vi "Main.vi"(7 "mode":T1) -> ()   [LabVIEW 2020, in "InstrumentStudioPlugin.lvlib"]
doc: "This template is for the Queued Message Handler design pattern.\n\nThe Event Handling Loop generates messages based on user interface actions.\n\nThe Message Handling Loop processes messages generated by the Event Handling Loop, or by other messages. The messages are string values, so new messages can be added easily to the Message Cases case structure in the Message Handling Loop. Each message cluster can also provide an optional value for Message Data, which is a variant that can be converted to whatever message-specific data is required."
uses:
  InstrumentStudioPlugin.lvlib
  controls/Plugin Mode.ctl
  InstrumentStudioPluginSDK.lvlibp/Plugin Events Enum.ctl
  controls/Configuration.ctl
  controls/Data.ctl
  Measurement Client Wrapper/Measurement Client Wrapper.lvclass
  controls/UI References.ctl
  Measurement Client Wrapper/Measurement Client Wrapper.lvclass/Measurement Client Wrapper.ctl
  Measurement Client Wrapper/Property/Read Display Name.vi
  Measurement Client Wrapper/Property/Read Version.vi
  subVIs/Message Queue/Enqueue Message (Single).vi
  subVIs/Message Queue/Enqueue Message (Array).vi
  <vilib>/Utility/error.llb/Error Cluster From Error Code.vi
  InstrumentStudioPluginSDK.lvlibp/Read Run Time Configuration.vi
  InstrumentStudioPluginSDK.lvlibp/Read Edit Time Configuration.vi
  InstrumentStudioPluginSDK.lvlibp/Write Run Time Configuration.vi
  InstrumentStudioPluginSDK.lvlibp/Write Edit Time Configuration.vi
  <vilib>/ErrorRing/Error Ring.xnode
  subVIs/Message Queue/Message Queue.lvlib
  subVIs/User Event - Stop/User Event - Stop.lvlib
  InstrumentStudioPluginSDK.lvlibp/Plugin Session.lvclass
  InstrumentStudioPluginSDK.lvlibp
panel:
  in  "Run Measurement":bool
  out "Version":string
  out "Measurement Name":string
  out "Status":string
  in  "Read Run Time Config":bool
  in  "Read Edit Time Config":bool
  in  "Session Id":u64
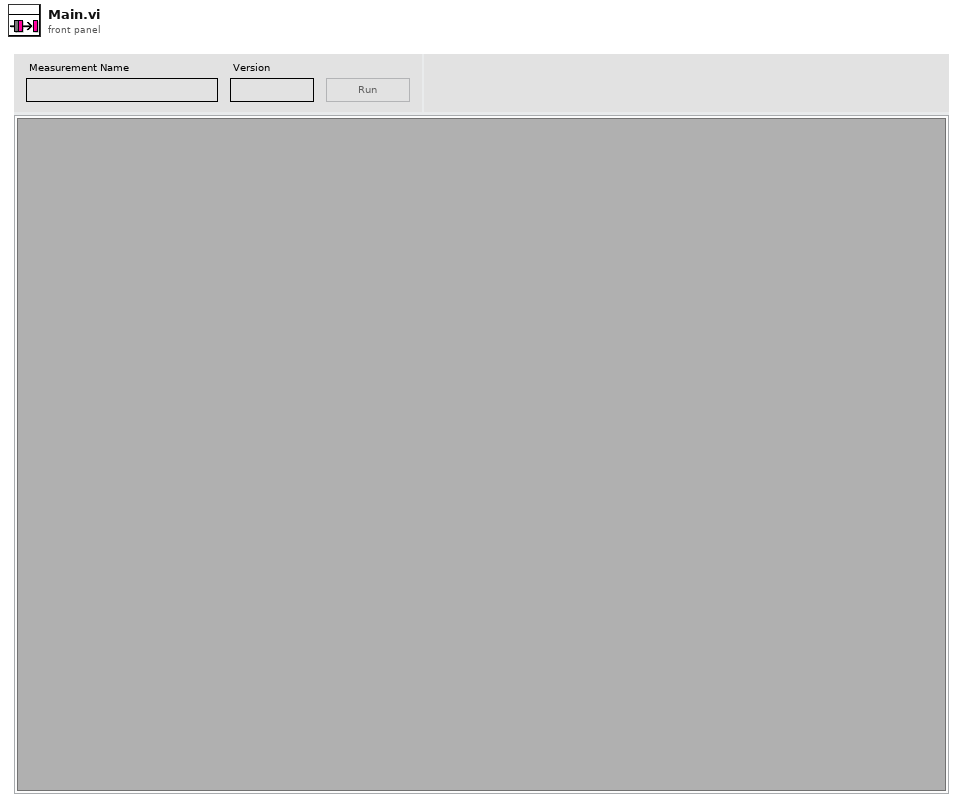
[diagram p1: front panel]
types:
  T1 = typedef "InstrumentStudioPlugin.lvlib/Plugin Mode.ctl" = enum16{"Interactive", "Automated"}
  T2 = typedef "InstrumentStudioPlugin.lvlib/UI References.ctl" = cluster{"UI Subpanel":refnum<vi>, "Status Message":string, "Matching UI & Meas Parameters?":bool}
  T3 = typedef "InstrumentStudioPlugin.lvlib/Data.ctl" = cluster{"Measurement Address":string, "Measurement Port":string, "Measurement Name":string, "Measurement Service":string, "Discovery Service address":string, "Measurement Service [obj]":refnum<class "Measurement Client Wrapper.lvclass">}
  T4 = typedef "InstrumentStudioPlugin.lvlib/Configuration.ctl" = cluster{"sample string":string}
  T5 = typedef "InstrumentStudioPluginSDK.lvlibp/Plugin Events Enum.ctl" = enum16{"Shutdown", "Project Saved", "Stop All Outputs"}
  T6 = typedef "InstrumentStudioPluginSDK.lvlibp/Event Registration Refnum.ctl" = refnum<event-registration>
  T7 = typedef "Message Queue.lvlib/All Message Queues.ctl" = cluster{"UI":refnum<queue>}
  T8 = cluster{"Event Refnum":T6, "Event Registration Refnum":refnum<event-registration>}
  T9 = enum8{"Enabled", "Disabled", "Disabled and Grayed Out"}
  T10 = cluster{"Measurement Name":string, "Measurement Service":string}
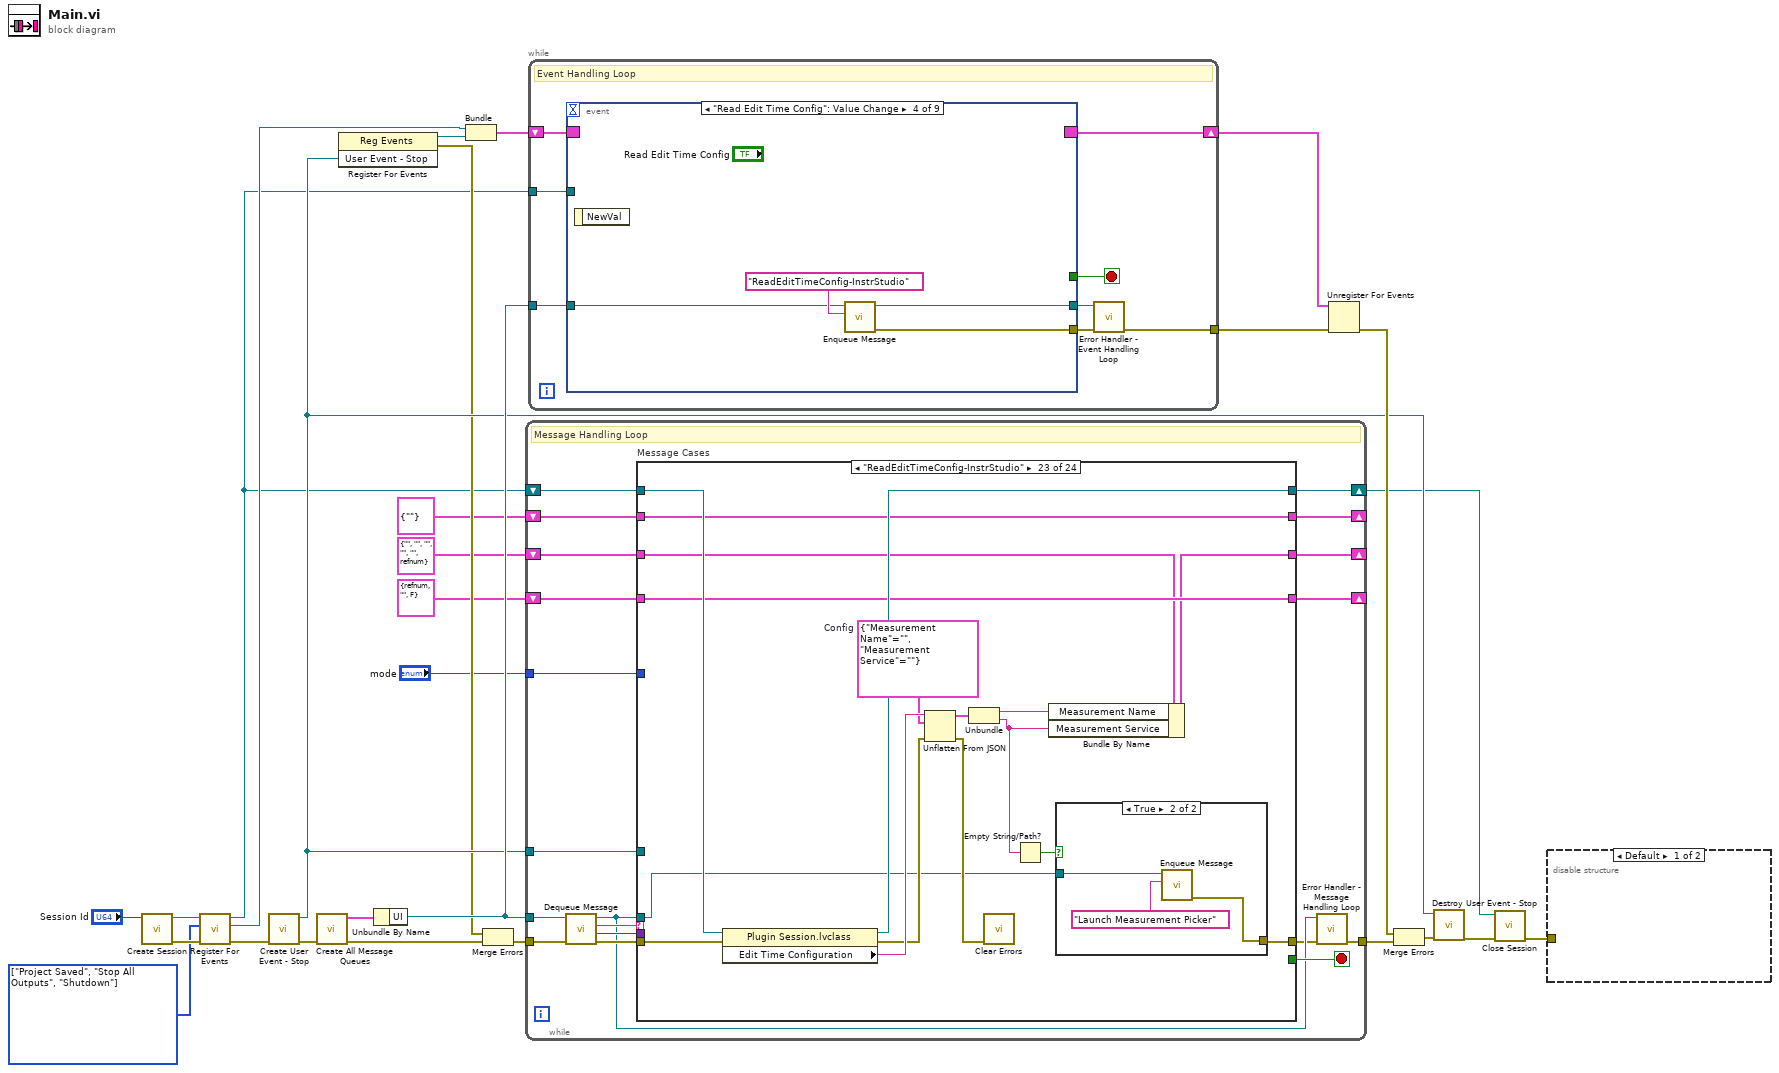
[diagram p0: block diagram]
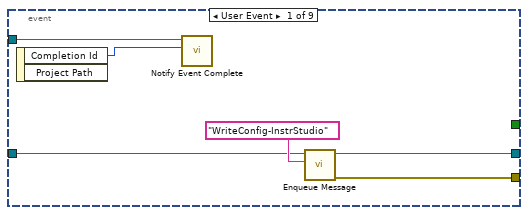
[diagram p3: hidden frame]
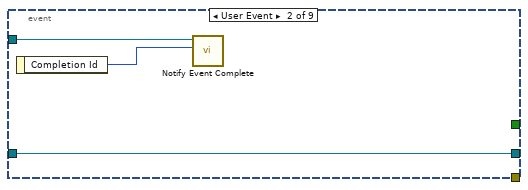
[diagram p4: hidden frame]
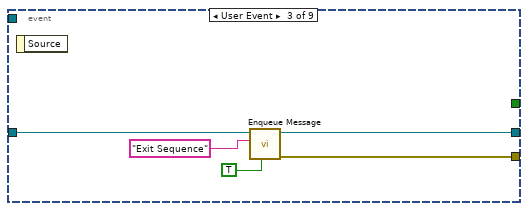
[diagram p5: hidden frame]
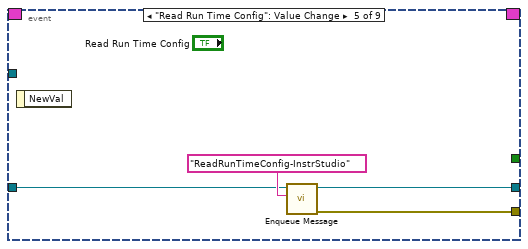
[diagram p6: hidden frame]
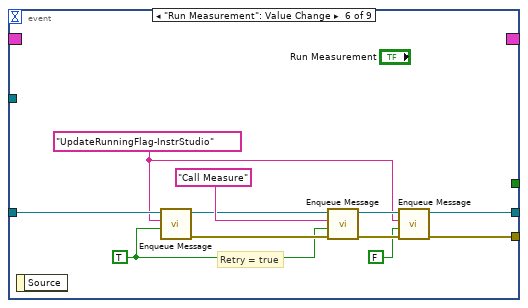
[diagram p7: hidden frame]
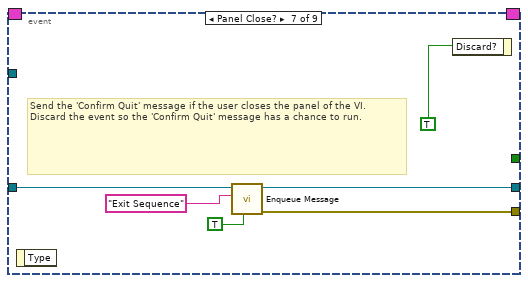
[diagram p8: hidden frame]
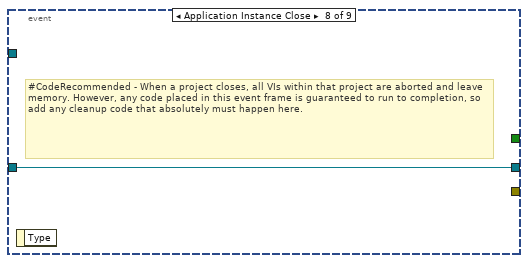
[diagram p9: hidden frame]
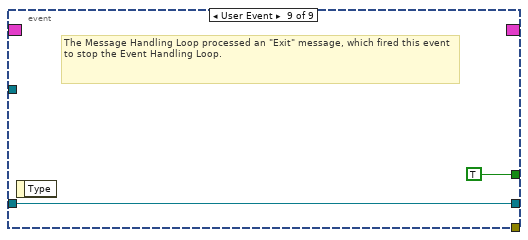
[diagram p10: hidden frame]
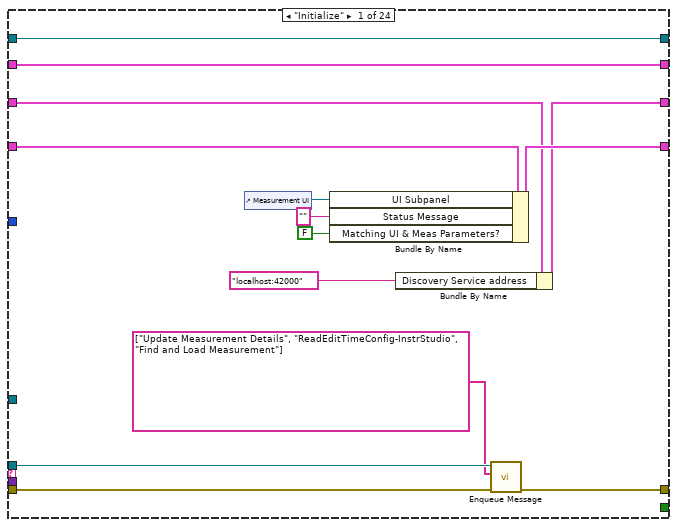
[diagram p11: hidden frame]
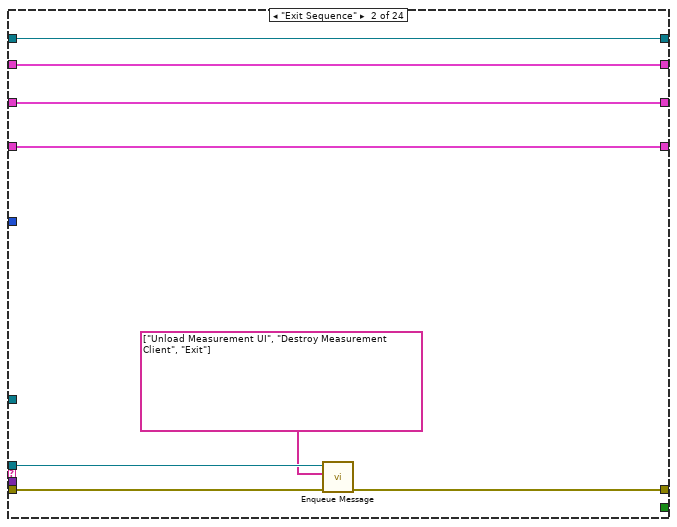
[diagram p12: hidden frame]
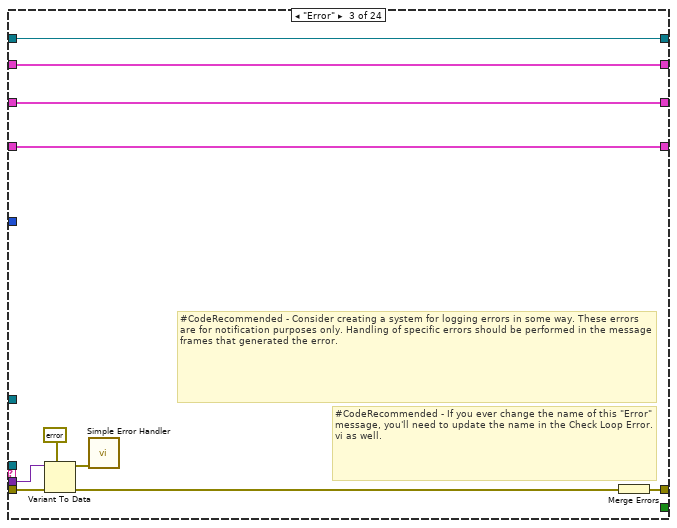
[diagram p13: hidden frame]
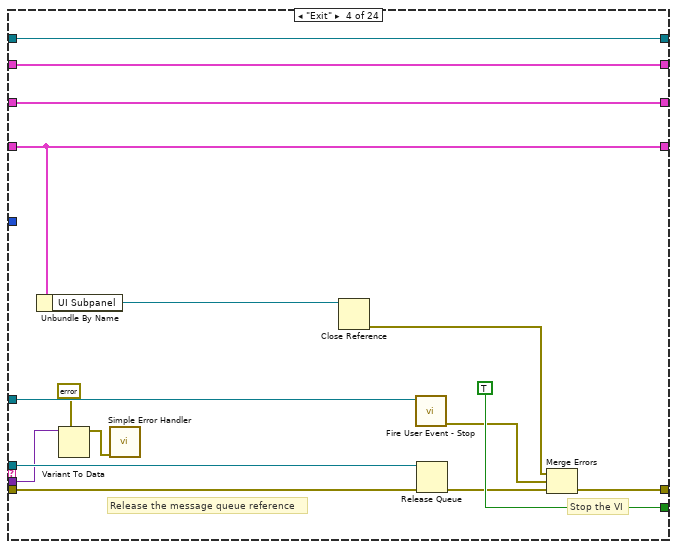
[diagram p14: hidden frame]
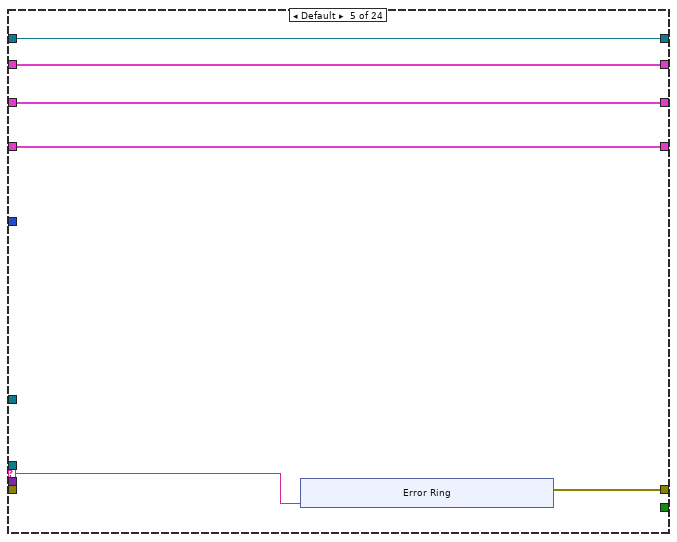
[diagram p15: hidden frame]
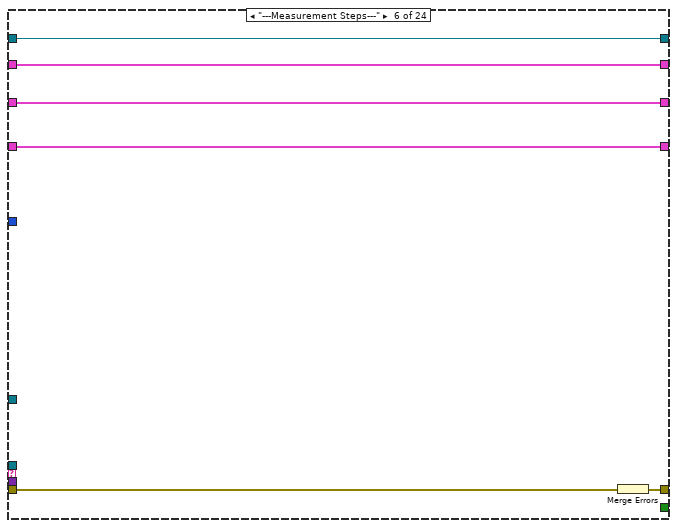
[diagram p16: hidden frame]
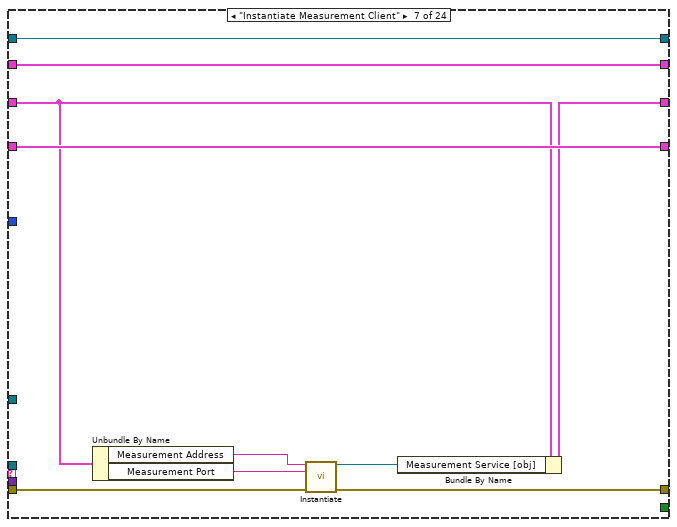
[diagram p17: hidden frame]
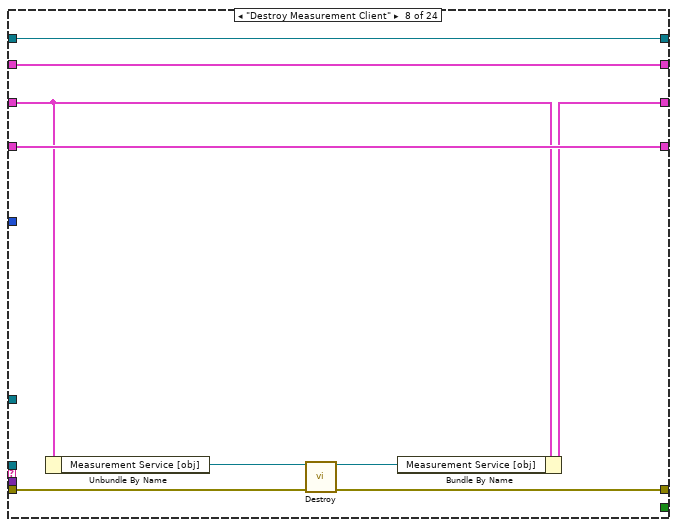
[diagram p18: hidden frame]
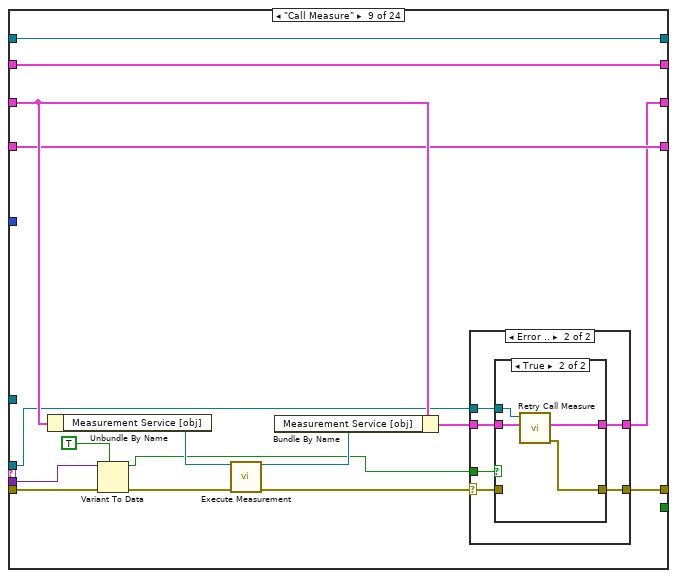
[diagram p19: hidden frame]
diagram:
  w12 = T5[] [enum."Project Saved", enum."Stop All Outputs", enum."Shutdown"] items=["Shutdown", "Project Saved", "Stop All Outputs"] ("Events To Register")
  n1 = call "Create Session.vi"("Session Id"="Session Id") -> ("error out"=w15:errorcluster, "Session out"=w13:refnum<class "Plugin Session.lvclass">)  [unwired: 6 in, 3 out]
  n2 = call "Register For Events.vi"("error in (no error)"=w15, "Events To Register"=w12, "Session in"=w13) -> ("error out"=w14:errorcluster, "Event Refnum"=w9:T6, "Session out"=w6:refnum<class "Plugin Session.lvclass">)  [unwired: 6 in]
  n3 = call "Create User Event - Stop.vi"("error in (no error)"=w14) -> ("error out"=w24:errorcluster, "User Event - Stop"=w19:refnum<user-event>)  [unwired: 9 in]
  n4 = call "Create All Message Queues.vi"("error in (no error)"=w24) -> ("error out"=w28:errorcluster, "Message Queues out"=w27:T7)  [unwired: 9 in]
  n5 = register-events(w19) -> (reference out=w11:refnum<event-registration>, error out=w17:errorcluster)  [unwired: 2 in]
  n6 = Unbundle By Name(w27) -> ("UI"=w25:refnum<queue>)
  n7 = Bundle("Event Refnum"=w9, "Event Registration Refnum"=w11) -> (w10:T8)  [unwired: 1 in]
  n8 = Merge Errors(w17, w28) -> (w18:errorcluster)
  n9 = while {
    tunnel: w25 -> [w39]
    shift-right: [w46] -> _
    shift-left: T3 {"Measurement Address"="", "Measurement Port"="", "Measurement Name"="", "Measurement Service"="", "Discovery Service address"="", "Measurement Service [obj]"=refnum} ("data") -> [w47]
    tunnel: w19 -> [w44]
    tunnel: w18 -> [w43]
    tunnel: [w37] -> w26
    shift-right: [w34] -> w8
    shift-left: w6 -> [w35]
    shift-right: [w33] -> _
    shift-left: T4 {"sample string"=""} ("Configuration") -> [w32]
    tunnel: "mode" -> [w31]
    shift-right: [w29] -> _
    shift-left: T2 {"UI Subpanel"=refnum, "Status Message"="", "Matching UI & Meas Parameters?"=FALSE} ("UI References") -> [w30]
    stop <- w45 stop-if-true
    # "Message Handling Loop"
    n10 = call "Dequeue Message.vi"("error in (no error)"=w43, "Message Queue"=w39) -> ("error out"=w42:errorcluster, "Message Data"=w40:variant, "Message"=w41:string, "dup Message Queue"=w38:refnum<queue>)  [unwired: 6 in]
    n11 = case "Message Cases" shown="\"ReadEditTimeConfig-InstrStudio\"" w41 {
      selector: w41 -> [_ _ _ _ w99 _ _ _ _ _ _ _ _ _ _ _ _ _ _ _ _ _ _ _]
      tunnel: w38 -> [w52 w63 _ w95 _ _ _ _ w141 _ _ _ w199 w220 _ _ _ _ _ _ _ _ w303 _]
      tunnel: w42 -> [w54 w65 w79 w88 _ w114 w121 w130 w138 w168 w178 w189 w201 w221 w229 w244 w255 w261 w276 w283 w292 w299 w316 w325]
      tunnel: [w53 w64 w73 w91 w100 w112 w120 w125 w142 w173 w177 w189 w197 w219 w229 w232 w254 w260 w274 w284 w290 w298 w302 w334] -> w36
      tunnel: w47 -> [w56 w69 w78 w94 w101 w113 w115 w127 w146 w171 w181 w188 w193 w218 w228 w245 w253 w264 w275 w287 w294 w297 w310 w330]
      tunnel: [w55 w69 w78 w94 w101 w113 w116 w128 w134 w172 w182 w188 w194 w217 w228 w245 w252 w268 w275 w287 w294 w297 w306 w330] -> w46
      tunnel: [_ _ _ TRUE _ _ _ _ _ _ _ _ _ _ _ _ _ _ _ _ _ _ _ _] -> w45
      tunnel: w40 -> [_ _ w77 w85 _ _ _ _ w139 _ _ _ _ _ _ _ _ _ _ w282 _ _ _ _]
      tunnel: w44 -> [_ _ _ w90 _ _ _ _ _ _ _ _ _ _ _ _ _ _ _ _ _ _ _ _]
      tunnel: w35 -> [w61 w68 w72 w84 w98 w111 w124 w133 w149 w175 w184 w187 w204 w224 w227 w247 w257 w270 w273 w286 w293 w301 w318 w336]
      tunnel: [w61 w68 w72 w84 w98 w111 w124 w133 w149 w175 w184 w187 w204 w224 w227 w247 w257 w270 w273 w285 w291 w300 w317 w335] -> w34
      tunnel: [w60 w67 w71 w83 w97 w110 w123 w132 w148 w174 w183 w186 w203 w223 w226 w246 w256 w269 w272 w278 w289 w296 w315 w332] -> w33
      tunnel: w32 -> [w60 w67 w71 w83 w97 w110 w123 w132 w148 w174 w183 w186 w203 w223 w226 w246 w256 w269 w272 w278 w289 w296 w315 w332]
      tunnel: w31 -> [_ _ _ _ _ _ _ _ _ _ _ _ _ _ _ _ _ _ _ _ _ _ _ _]
      tunnel: w30 -> [w59 w66 w70 w82 w96 w109 w122 w131 w144 w170 w180 w185 w202 w222 w225 w237 w251 w267 w271 w277 w288 w295 w314 w331]
      tunnel: [w57 w66 w70 w82 w96 w109 w122 w131 w144 w169 w180 w185 w202 w222 w225 w237 w251 w265 w271 w277 w288 w295 w314 w331] -> w29
      frame "Initialize" {
        # "Initialize - All initialization work should take place in this message, since other loops can potentially enqueue messages that execute immediately after this one."
        n12 = control-ref of="Measurement UI"() -> (w58:refnum<vi>)
        n13 = Bundle By Name(cluster=w59, "UI Subpanel"=w58, "Status Message"="", "Matching UI & Meas Parameters?"=FALSE) -> (w57:T2)
        n14 = Bundle By Name(cluster=w56, "Discovery Service address"="localhost:42000") -> (w55:T3)
        n15 = call-poly "Enqueue Message.vi"("error in (no error)"=w54, "Message Array"=string[] ["Update Measurement Details", "ReadEditTimeConfig-InstrStudio", "Find and Load Measurement"], "Message Queue"=w52) -> ("error out"=w53:errorcluster)  [unwired: 7 in, 1 out]
      }
      frame "Exit Sequence" {
        n16 = call-poly "Enqueue Message.vi"("error in (no error)"=w65, "Message Array"=string[] ["Unload Measurement UI", "Destroy Measurement Client", "Exit"], "Message Queue"=w63) -> ("error out"=w64:errorcluster)  [unwired: 7 in, 1 out]
      }
      frame "Error" {
        # "#CodeRecommended - If you ever change the name of this \"Error\" message, you'll need to update the name in the Check Loop Error.vi as well."
        # "#CodeRecommended - Consider creating a system for logging errors in some way. These errors are for notification purposes only. Handling of specific errors should be performed in the message frames that generated the error."
        # "Error - Display an error dialog. This message is sent by the \"Error Handler\" VIs at the end of other loops in this application."
        n17 = Variant To Data(error in=w79, type=errorcluster {"status"=FALSE, "code"=0, "source"=""} ("error constant"), Variant=w77) -> (data=w75:errorcluster, error out=w74:errorcluster)
        n18 = call <vilib>:"Simple Error Handler.vi"("error in (no error)"=w75) -> ()  [unwired: 4 in, 5 out]
        n19 = Merge Errors(w74) -> (w73:errorcluster)
      }
      frame "Exit" {
        # "Stop the VI"
        # "Release the message queue reference"
        # "Exit - Exit the application."
        n20 = Unbundle By Name(w82) -> ("UI Subpanel"=w81:refnum<vi>)
        n21 = Variant To Data(type=errorcluster {"status"=FALSE, "code"=0, "source"=""} ("error constant"), Variant=w85) -> (data=w86:errorcluster)  [unwired: 1 in, 1 out]
        n22 = call <vilib>:"Simple Error Handler.vi"("error in (no error)"=w86) -> ()  [unwired: 4 in, 5 out]
        n23 = Close Reference(reference=w81) -> (error out=w80:errorcluster)  [unwired: 1 in]
        n24 = call "Fire User Event - Stop.vi"("User Event - Stop"=w90) -> ("error out"=w89:errorcluster)  [unwired: 10 in]
        n25 = Release Queue(queue=w95, error in (no error)=w88) -> (error out=w92:errorcluster)  [unwired: 1 in, 2 out]
        n26 = Merge Errors(w80, w89, w92) -> (w91:errorcluster)
      }
      frame Default {
        # "'Default' case only runs if there is a message that isn't defined in any of the other cases.  Output a programming error."
        n27 = xnode "Error Ring"("parameter 0"=w99) -> ("error out"=w100:errorcluster)
      }
      frame "---Measurement Steps---" {
        # "Duplicate this frame when creating new messages.  Change this comment in the duplicated frame to describe this message."
        n28 = Merge Errors(w114) -> (w112:errorcluster)
      }
      frame "Instantiate Measurement Client" {
        n29 = Unbundle By Name(w115) -> ("Measurement Address"=w119:string, "Measurement Port"=w118:string)
        n30 = call "Instantiate.vi"("location"=w119, "insecurePort"=w118, "error in (no error)"=w121) -> ("Measurement Client Wrapper out"=w117:refnum<class "Measurement Client Wrapper.lvclass">, "error out"=w120:errorcluster)  [unwired: 11 in]
        n31 = Bundle By Name(cluster=w115, "Measurement Service [obj]"=w117) -> (w116:T3)
      }
      frame "Destroy Measurement Client" {
        n32 = Unbundle By Name(w127) -> ("Measurement Service [obj]"=w126:refnum<class "Measurement Client Wrapper.lvclass">)
        n33 = call "Destroy.vi"("Measurement Client Wrapper in"=w126, "error in"=w130) -> ("Measurement Client Wrapper out"=w129:refnum<class "Measurement Client Wrapper.lvclass">, "error out"=w125:errorcluster)  [unwired: 12 in]
        n34 = Bundle By Name(cluster=w127, "Measurement Service [obj]"=w129) -> (w128:T3)
      }
      frame "Call Measure" {
        n35 = Unbundle By Name(w146) -> ("Measurement Service [obj]"=w147:refnum<class "Measurement Client Wrapper.lvclass">)
        n36 = Variant To Data(error in=w138, type=TRUE, Variant=w139) -> (data=w136:bool, error out=w137:errorcluster)
        n37 = call "Execute Measurement.vi"("Measurement Client Wrapper"=w147, "error in"=w137) -> ("Measurement Client Wrapper out"=w145:refnum<class "Measurement Client Wrapper.lvclass">, "error out"=w143:errorcluster)  [unwired: 12 in]
        n38 = Bundle By Name(cluster=w146, "Measurement Service [obj]"=w145) -> (w135:T3)
        n39 = case shown="Error .." w143 {
          selector: w143 -> [w151 w154]
          tunnel: [w151 w156] -> w142
          tunnel: w141 -> [_ w157]
          tunnel: w136 -> [_ w155]
          tunnel: w135 -> [w150 w153]
          tunnel: [w150 w152] -> w134
          frame No Error {
          }
          frame Error {
            n40 = case shown="True" w155 {
              tunnel: w157 -> [_ w163]
              tunnel: [w159 w162] -> w156
              tunnel: w154 -> [w159 _]
              tunnel: w153 -> [w158 w161]
              tunnel: [w158 w160] -> w152
              frame False {
              }
              frame True {
                n41 = call "Retry Call Measure.vi"("Data In"=w161, "Message Queue"=w163) -> ("error out"=w162:errorcluster, "data out"=w160:T3)  [unwired: 7 in, 1 out]
              }
            }
          }
        }
      }
      frame "Verify UI-Measurement Parameters" {
        n42 = Unbundle By Name(w171) -> ("Measurement Service [obj]"=w167:refnum<class "Measurement Client Wrapper.lvclass">)
        n43 = call "LabVIEW Measurement UI - Verify Parameter Matching.vi"("Measurement Client Wrapper in"=w167, "error in"=w168) -> ("Measurement Client Wrapper"=w166:refnum<class "Measurement Client Wrapper.lvclass">, "Status"=w165:string, "Matching?"=w164:bool, "error out"=w173:errorcluster)  [unwired: 10 in]
        n44 = Bundle By Name(cluster=w171, "Measurement Service [obj]"=w166) -> (w172:T3)
        n45 = Bundle By Name(cluster=w170, "Status Message"=w165, "Matching UI & Meas Parameters?"=w164) -> (w169:T2)
      }
      frame "Update UI Default Values" {
        n46 = Unbundle By Name(w181) -> ("Measurement Service [obj]"=w179:refnum<class "Measurement Client Wrapper.lvclass">)
        n47 = call "Update Any Values to UI.vi"("Measurement Client Wrapper"=w179, "error in"=w178) -> ("Measurement Client Wrapper out"=w176:refnum<class "Measurement Client Wrapper.lvclass">, "error out"=w177:errorcluster)  [unwired: 12 in]
        n48 = Bundle By Name(cluster=w181, "Measurement Service [obj]"=w176) -> (w182:T3)
      }
      frame "------Front Panel Interaction------" {
      }
      frame "Launch Measurement Picker" {
        n49 = Unbundle By Name(w193) -> ("Discovery Service address"=w192:string)
        n50 = call "Measurement Picker.vi"("discovery address"=w192, "error in"=w201) -> ("Cancelled?"=w200:bool, "Measurement location"=w196:string, "Measurement port"=w195:string, "Measurement Name"=w190:string, "Measurement Service"=w191:string, "error out"=w198:errorcluster)  [unwired: 8 in]
        n51 = case shown="False" w200 {
          tunnel: w199 -> [w214 _]
          tunnel: w198 -> [w213 w216]
          tunnel: [w212 w216] -> w197
          tunnel: w196 -> [w210 _]
          tunnel: w195 -> [w209 _]
          tunnel: w193 -> [w211 w215]
          tunnel: [w208 w215] -> w194
          tunnel: w191 -> [w206 _]
          tunnel: w190 -> [w205 _]
          frame False {
            n52 = Bundle By Name(cluster=w211, "Measurement Address"=w210, "Measurement Port"=w209, "Measurement Service"=w206, "Measurement Name"=w205) -> (w208:T3)
            n53 = call-poly "Enqueue Message.vi"("error in (no error)"=w213, "Message Array"=string[] ["Update Measurement Details", "Unload Measurement UI", "Destroy Measurement Client", "Instantiate Measurement Client", "Load Measurement UI", "Verify UI-Measurement Parameters", "Update UI Default Values", "Update Measurement Details", "WriteConfig-InstrStudio"], "Message Queue"=w214) -> ("error out"=w212:errorcluster)  [unwired: 7 in, 1 out]
          }
          frame True {
          }
        }
      }
      frame "Find and Load Measurement" {
        n54 = call "Find And Load Measurement.vi"("error in (no error)"=w221, "data in"=w218, "Message Queue"=w220) -> ("error out"=w219:errorcluster, "data out"=w217:T3)  [unwired: 6 in, 1 out]
      }
      frame "------Front Panel Updates------" {
      }
      frame "Update Measurement Details" {
        n55 = Unbundle By Name(w237) -> ("Status Message"=→"Status":string, "Matching UI & Meas Parameters?"=w230:bool)
        n56 = Unbundle By Name(w245) -> ("Measurement Service [obj]"=w235:refnum<class "Measurement Client Wrapper.lvclass">)
        n57 = Select(t=T9."Enabled" ("Disabled"), s=w230, f=T9."Disabled and Grayed Out" ("Disabled")) -> (s? t:f=w241:T9)
        n58 = property class="Measurement Client Wrapper.lvcl"(reference=w235) -> (error out=w231:errorcluster, "Property:Display Name"=→"Measurement Name":string, "Property:Version"=→"Version":string)  [unwired: 1 in, 1 out]
        n59 = property on="Run Measurement" class="Bool"(error in=w244, "DisabledEnum"=w241) -> (error out=w240:errorcluster)  [unwired: 1 in, 1 out]
        n60 = Not(x=w230) -> (.not. x?=w238:bool)
        n61 = property on="Status" class="Str"(error in=w240, "Visible"=w238) -> (error out=w239:errorcluster)  [unwired: 1 in, 1 out]
        n62 = Merge Errors(w239, w231) -> (w232:errorcluster)
      }
      frame "Load Measurement UI" {
        n63 = Unbundle By Name(w253) -> ("Measurement Service [obj]"=w249:refnum<class "Measurement Client Wrapper.lvclass">)
        n64 = Unbundle By Name(w251) -> ("UI Subpanel"=w248:refnum<vi>)
        n65 = call "LabVIEW Measurement UI - Open & Run.vi"("error in"=w255, "UI Subpanel"=w248, "Measurement Client Wrapper in"=w249) -> ("error out"=w254:errorcluster, "Measurement Client Wrapper"=w250:refnum<class "Measurement Client Wrapper.lvclass">)  [unwired: 6 in, 1 out]
        n66 = Bundle By Name(cluster=w253, "Measurement Service [obj]"=w250) -> (w252:T3)
      }
      frame "Unload Measurement UI" {
        n67 = Unbundle By Name(w264) -> ("Measurement Service [obj]"=w263:refnum<class "Measurement Client Wrapper.lvclass">)
        n68 = Unbundle By Name(w267) -> ("UI Subpanel"=w259:refnum<vi>)
        n69 = call "LabVIEW Measurement UI - Stop & Close.vi"("error in"=w261, "UI Subpanel"=w259, "Measurement Client Wrapper in"=w263) -> ("error out"=w260:errorcluster, "Measurement Client Wrapper"=w262:refnum<class "Measurement Client Wrapper.lvclass">)  [unwired: 7 in]
        n70 = Bundle By Name(cluster=w267, "Matching UI & Meas Parameters?"=FALSE, "Status Message"="") -> (w265:T2)
        n71 = Bundle By Name(cluster=w264, "Measurement Service [obj]"=w262) -> (w268:T3)
      }
      frame "---Instrument Studio Interaction---" {
        # "Duplicate this frame when creating new messages.  Change this comment in the duplicated frame to describe this message."
        n72 = Merge Errors(w276) -> (w274:errorcluster)
      }
      frame "UpdateRunningFlag-InstrStudio" {
        n73 = Variant To Data(error in=w283, type=TRUE, Variant=w282) -> (data=w280:bool, error out=w279:errorcluster)
        n74 = call "Update Running State.vi"("error in (no error)"=w279, "Is Running"=w280, "Plugin Session in"=w286) -> ("error out"=w284:errorcluster, "Plugin Session out"=w285:refnum<class "Plugin Session.lvclass">)  [unwired: 7 in]
      }
      frame "ReadISProjectPath" {
        n75 = call "Read Project Path.vi"("error in (no error)"=w292, "Session in"=w293) -> ("error out"=w290:errorcluster, "Session out"=w291:refnum<class "Plugin Session.lvclass">)  [unwired: 7 in, 1 out]
      }
      frame "ReadRunTimeConfig-InstrStudio" {
        n76 = property class="Plugin Session.lvclass" props=["Run Time Configuration"](reference=w301, error in=w299) -> (reference out=w300:refnum<class "Plugin Session.lvclass">, error out=w298:errorcluster)  [unwired: 1 out]
      }
      frame "ReadEditTimeConfig-InstrStudio" {
        w311 = T10 {"Measurement Name"="", "Measurement Service"=""}  # Config
        n77 = property class="Plugin Session.lvclass"(reference=w318, error in=w316) -> (reference out=w317:refnum<class "Plugin Session.lvclass">, error out=w312:errorcluster, "Edit Time Configuration"=w313:string)
        n78 = Unflatten From JSON(JSON string=w313, type and defaults=w311, error in (no error)=w312) -> (value=w309:T10, error out=w307:errorcluster)  [unwired: 4 in]
        n79 = Unbundle(w309) -> ("Measurement Name"=w308:string, "Measurement Service"=w305:string)
        n80 = call <vilib>:"Clear Errors.vi"("error in (no error)"=w307) -> ()  [unwired: 5 in, 2 out]
        n81 = Empty String/Path?(string/path=w305) -> (empty?=w304:bool)
        n82 = Bundle By Name(cluster=w310, "Measurement Name"=w308, "Measurement Service"=w305) -> (w306:T3)
        n83 = case shown="True" w304 {
          tunnel: w303 -> [_ w322]
          tunnel: [errorcluster {"status"=FALSE, "code"=0, "source"=""} ("error out") w320] -> w302
          frame False {
          }
          frame True {
            n84 = call-poly "Enqueue Message.vi"("Message"="Launch Measurement Picker", "Message Queue"=w322) -> ("error out"=w320:errorcluster)  [unwired: 8 in, 1 out]
          }
        }
      }
      frame "WriteConfig-InstrStudio" {
        w326 = T10 {"Measurement Name"="", "Measurement Service"=""}  # Config
        n85 = Unbundle By Name(w330) -> ("Measurement Name"=w329:string, "Measurement Service"=w328:string)
        n86 = Bundle(cluster=w326, "Measurement Name"=w329, "Measurement Service"=w328) -> (w327:T10)
        n87 = Flatten To JSON(anything=w327, error in (no error)=w325) -> (JSON string=w323:string, 11:w324:errorcluster)  [unwired: 1 in]
        n88 = property class="Plugin Session.lvclass"(reference=w336, error in=w324, "Run Time Configuration"="", "Edit Time Configuration"=w323) -> (reference out=w335:refnum<class "Plugin Session.lvclass">, error out=w334:errorcluster)
      }
    }
    n89 = call "Error Handler - Message Handling Loop.vi"("error in (no error)"=w36, "Message Queue"=w38) -> ("dup error in"=w37:errorcluster)  [unwired: 8 in, 1 out]
  }
  n90 = while {
    tunnel: w25 -> [w344]
    shift-right: [w342] -> w21
    shift-left: w10 -> [w343]
    tunnel: [w338] -> w20
    tunnel: w6 -> [w337]
    stop <- w340 stop-if-true
    # "Event Handling Loop"
    n91 = event shown="[3] \"Read Edit Time Config\": Value Change" {
      selector: w343 -> [_ _ _ _ _ _ _ _ _]
      dyn-events: [_ _ _ _ _ _ _ _ _] -> w342
      timeout: _ -> [_ _ _ _ _ _ _ _ _]
      tunnel: [_ _ _ _ _ _ _ _ TRUE ("Discard?")] -> w340
      tunnel: w344 -> [w347 w353 w356 w361 w365 w376 w382 w384 w386]
      tunnel: [w345 _ w354 w359 w363 w371 w381 _ _] -> w341
      tunnel: [w346 w353 w355 w360 w364 w370 w380 w384 w386] -> w339
      tunnel: w337 -> [w350 w352 _ _ _ _ _ _ _]
      event User Event {
        n92 = event-data() -> ("Completion Id"=w349:i64)  [unwired: 1 in, 1 out]
        n93 = call "Notify Event Complete.vi"("Completion Id"=w349, "Session in"=w350) -> ()  [unwired: 8 in, 2 out]
        n94 = call-poly "Enqueue Message.vi"("Message"="WriteConfig-InstrStudio", "Message Queue"=w347) -> ("error out"=w345:errorcluster, "dup Message Queue"=w346:refnum<queue>)  [unwired: 8 in]
      }
      event User Event {
        n95 = event-data() -> ("Completion Id"=w351:i64)  [unwired: 1 in]
        n96 = call "Notify Event Complete.vi"("Completion Id"=w351, "Session in"=w352) -> ()  [unwired: 8 in, 2 out]
      }
      event User Event {
        n97 = event-data() -> ()  [unwired: 1 in, 1 out]
        n98 = call-poly "Enqueue Message.vi"("Priority Message? (F)"=TRUE, "Message"="Exit Sequence", "Message Queue"=w356) -> ("error out"=w354:errorcluster, "dup Message Queue"=w355:refnum<queue>)  [unwired: 7 in]
      }
      event "Read Edit Time Config": Value Change {
        n99 = event-data() -> ()  [unwired: 1 in, 1 out]
        n100 = call-poly "Enqueue Message.vi"("Message"="ReadEditTimeConfig-InstrStudio", "Message Queue"=w361) -> ("error out"=w359:errorcluster, "dup Message Queue"=w360:refnum<queue>)  [unwired: 8 in]
      }
      event "Read Run Time Config": Value Change {
        n101 = event-data() -> ()  [unwired: 1 in, 1 out]
        n102 = call-poly "Enqueue Message.vi"("Message"="ReadRunTimeConfig-InstrStudio", "Message Queue"=w365) -> ("error out"=w363:errorcluster, "dup Message Queue"=w364:refnum<queue>)  [unwired: 8 in]
      }
      event "Run Measurement": Value Change {
        w367 = TRUE
        w369 = "UpdateRunningFlag-InstrStudio" ("Message")
        # "Retry = true"
        n103 = event-data() -> ()  [unwired: 1 in, 1 out]
        n104 = call-poly "Enqueue Message.vi"("Message Data"=w367, "Message"=w369, "Message Queue"=w376) -> ("error out"=w374:errorcluster, "dup Message Queue"=w375:refnum<queue>)  [unwired: 7 in]
        n105 = call-poly "Enqueue Message.vi"("error in (no error)"=w374, "Message Data"=w367, "Message"="Call Measure", "Message Queue"=w375) -> ("error out"=w372:errorcluster, "dup Message Queue"=w373:refnum<queue>)  [unwired: 6 in]
        n106 = call-poly "Enqueue Message.vi"("error in (no error)"=w372, "Message Data"=FALSE, "Message"=w369, "Message Queue"=w373) -> ("error out"=w371:errorcluster, "dup Message Queue"=w370:refnum<queue>)  [unwired: 6 in]
      }
      event Panel Close? {
        # "Send the 'Confirm Quit' message if the user closes the panel of the VI. Discard the event so the 'Confirm Quit' message has a chance to run."
        n107 = event-data() -> ()  [unwired: 1 in, 1 out]
        n108 = call-poly "Enqueue Message.vi"("Priority Message? (F)"=TRUE, "Message"="Exit Sequence", "Message Queue"=w382) -> ("error out"=w381:errorcluster, "dup Message Queue"=w380:refnum<queue>)  [unwired: 7 in]
        n109 = event-data("Discard?"=TRUE) -> ()  [unwired: 1 in, 1 out]
      }
      event Application Instance Close {
        # "#CodeRecommended - When a project closes, all VIs within that project are aborted and leave memory. However, any code placed in this event frame is guaranteed to run to completion, so add any cleanup code that absolutely must happen here."
        n110 = event-data() -> ()  [unwired: 1 in, 1 out]
      }
      event User Event {
        # "The Message Handling Loop processed an \"Exit\" message, which fired this event to stop the Event Handling Loop."
        n111 = event-data() -> ()  [unwired: 1 in, 1 out]
      }
    }
    n112 = call "Error Handler - Event Handling Loop.vi"("error in (no error)"=w341, "Message Queue"=w339) -> ("dup error in"=w338:errorcluster)  [unwired: 8 in, 1 out]
  }
  n113 = Unregister For Events(event registration refnum=w21, error in=w20) -> (error out=w22:errorcluster)
  n114 = Merge Errors(w22, w26) -> (w23:errorcluster)
  n115 = call "Destroy User Event - Stop.vi"("error in (no error)"=w23, "User Event - Stop"=w19) -> ("error out"=w7:errorcluster)  [unwired: 9 in]
  n116 = call "Close Session.vi"("error in (no error)"=w7, "Session in"=w8) -> ("error out"=w1:errorcluster)  [unwired: 9 in]
  n117 = disable-structure shown="Default" {
    disable-tunnel: w1 -> [_ _]
    frame condition #0 (active) {
    }
    frame condition #1 {
      # "Call Quit LabVIEW if running as a built application."
    }
  }
